vi "adjustScanPiezoZ.vi"() -> ()   [LabVIEW 2014]
uses:
  <userlib>/Nanonis Prog Interface V5/Nanonis Prog Interface.lvlib
panel:
  out "Z position (m)":sgl format="%#_6p"
  in  "z position":sgl
  in  "milliseconds to wait":u32
  in  "Direction":enum16{"X +", "X -", "Y +", "Y -", "Z +", "Z -"}(ring)=enum."Z -"
  in  "Amplitude (V) (NaN=no change)":sgl=nan
  in  "Frequency (Hz) (NaN=no change)":sgl=nan
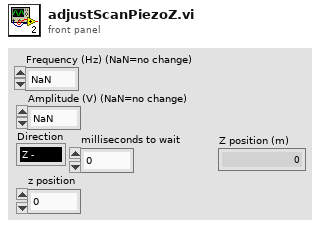
[diagram p1: front panel]
types:
  T1 = enum8{"Group 1", "Group 2", "Group 3", "Group 4", "Group 5", "Group 6"}
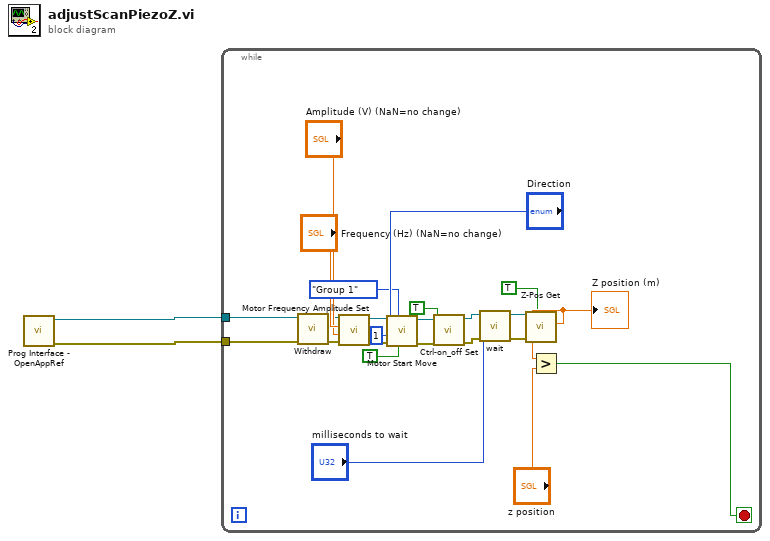
[diagram p0: block diagram]
diagram:
  n1 = call <userlib>:"Prog Interface - OpenAppRef.vi"() -> ("Error out"=w2:errorcluster, "Application reference"=w1:refnum<vi>)  [unwired: 6 in]
  n2 = while {
    tunnel: w2 -> [w26]
    tunnel: w1 -> [w25]
    stop <- w3 stop-if-true
    n3 = call <userlib>:"Withdraw.vi"("Error in (no error)"=w26, "Application ref in"=w25) -> ("Error out"=w19:errorcluster, "Application ref out"=w18:refnum<vi>)  [unwired: 8 in]
    n4 = call <userlib>:"Motor Frequency Amplitude Set.vi"("Error in (no error)"=w19, "Amplitude (V) (NaN=no change)"="Amplitude (V) (NaN=no change)", "Frequency (Hz) (NaN=no change)"="Frequency (Hz) (NaN=no change)", "Application ref in"=w18) -> ("Error out"=w17:errorcluster, "Application ref out"=w16:refnum<vi>)  [unwired: 6 in]
    n5 = call <userlib>:"Motor Start Move.vi"("Wait until finished? (F)"=TRUE, "Group"=T1."Group 1", "Error in (no error)"=w17, "Number of steps"=u16 1, "Direction"="Direction", "Application ref in"=w16) -> ("Error out"=w12:errorcluster, "Application ref out"=w11:refnum<vi>)  [unwired: 3 in]
    n6 = call <userlib>:"Ctrl-on_off Set.vi"("error in (no error)"=w12, "Z Controller ON/OFF"=TRUE, "Application ref in"=w11) -> ("error out"=w8:errorcluster, "Application ref out"=w10:refnum<vi>)  [unwired: 7 in]
    n7 = call "wait.vi"("error in"=w8, "milliseconds to wait"="milliseconds to wait", "application reference in"=w10) -> ("error out"=w7:errorcluster, "application reference out"=w6:refnum<vi>)  [unwired: 7 in]
    n8 = call <userlib>:"Z-Pos Get.vi"("Wait for newest data (F=False)"=TRUE, "error in (no error)"=w7, "Application ref in"=w6) -> ("Z position (m)"=w5:sgl)  [unwired: 6 in, 2 out]
    "Z position (m)" <- w5
    n9 = Greater?(x=w5, y="z position") -> (0:w3:bool)
  }
